vi "GetAbstractClassPath.vi"(0 "instrument_type_id":string, 11 "error in (no error)":errorcluster) -> (4 "appended path":path, 15 "error out":errorcluster)   [LabVIEW 2020, in "DMMFactory.lvlib" / "DMMFactory.lvclass"]
uses:
  DMMFactory.lvclass
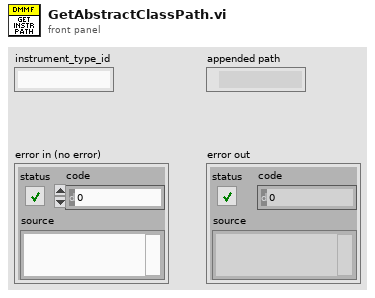
[diagram p1: front panel]
types:
  T1 = typedef "DMMFactory.lvlib/DMMFactory.lvclass/DMM_Factory_Paths.ctl" = cluster{"AbstarctClasses":path, "InstrMappingConfig":path}
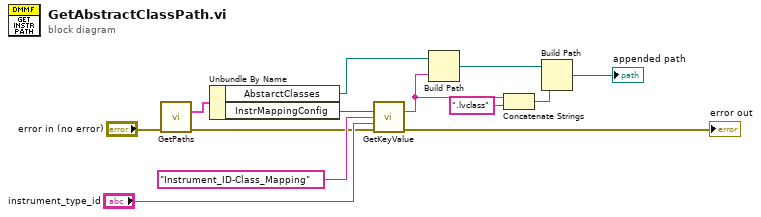
[diagram p0: block diagram]
diagram:
  n1 = call "GetPaths.vi"("error in"="error in (no error)") -> ("DDMM_Factory_Paths"=w3:T1, "error out"=w2:errorcluster)  [unwired: 13 in]
  n2 = Unbundle By Name(w3) -> ("AbstarctClasses"=w8:path, "InstrMappingConfig"=w5:path)
  n3 = call "GetKeyValue.vi"("ConfigurationFilePath"=w5, "Section"="Instrument_ID-Class_Mapping", "Key"="instrument_type_id", "error in"=w2) -> ("Value"=w10:string, "error out"=→"error out":errorcluster)  [unwired: 10 in]
  n4 = Build Path(base path=w8, name or relative path=w10) -> (appended path=w9:path)
  n5 = Concatenate Strings(w10, ".lvclass" ("string")) -> (w11:string)
  n6 = Build Path(base path=w9, name or relative path=w11) -> (appended path=→"appended path":path)
